vi "initialise.vi"(8 "error in (no error)":errorcluster, 11 "DAQ_DL091205Readers in":refnum<class "DAQ_DL091205Readers.lvclass">) -> (0 "error out":errorcluster, 3 "DAQ_DL091205Readers out":refnum<class "DAQ_DL091205Readers.lvclass">)   [LabVIEW 2010, in "DAQ_DL091205Readers.lvclass"]
doc: "The dynamic dispatch-version of this VI initalises the plug-in object by allocating and initalising any dynamic resources need."
uses:
  DAQ_DL091205Readers.lvclass
  DAQ_DL090211Scaffold/DAQ_DL090211Scaffold/DAQ_DL090211Scaffold.lvclass
  DAQ_DL091205Readers.lvclass/DAQ_DL091205Readers.ctl
  SignalReader/GenericSignalReader/GenericSignalReader/GenericSignalReader.lvclass
  common/classes/ErrorController/ErrorController/class_data.vi
  common/classes/ErrorController/ErrorController/ErrorController.lvclass
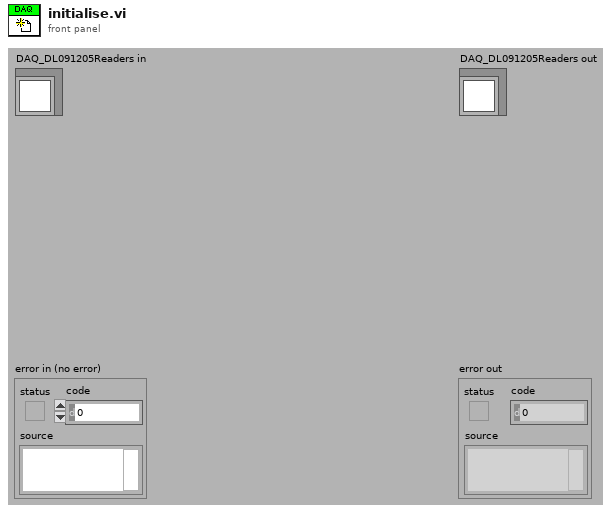
[diagram p1: front panel]
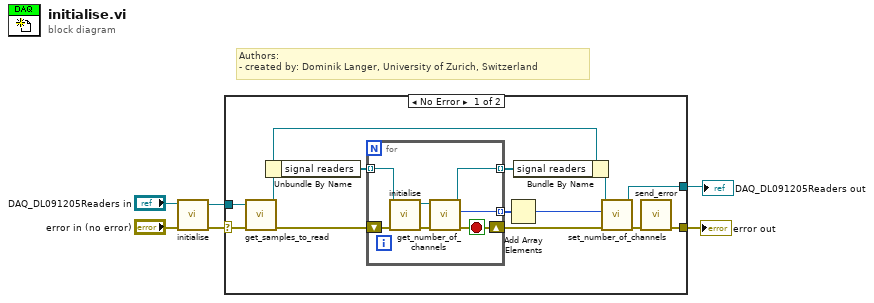
[diagram p0: block diagram]
diagram:
  # "Authors: \n- created by: Dominik Langer, University of Zurich, Switzerland"
  n1 = call-parent "initialise.vi"("error in (no error)"="error in (no error)", "GenericPlugin in"="DAQ_DL091205Readers in") -> ("error out"=w4:errorcluster, "GenericPlugin out"=w3:refnum<class "DAQ_DL091205Readers.lvclass">)  [unwired: 8 in]
  n2 = case shown="No Error" w4 {
    selector: w4 -> [w15 w27]
    tunnel: [w13 w27] -> w2
    tunnel: w3 -> [w17 w28]
    tunnel: [w8 w28] -> w1
    frame No Error {
      n3 = call-dynamic "get_samples_to_read.vi"("error in (no error)"=w15, "GenericDAQ.lvclass in"=w17) -> ("error out"=w14:errorcluster, "GenericDAQ.lvclass out"=w16:refnum<class "DAQ_DL091205Readers.lvclass">)  [unwired: 7 in, 1 out]
      n4 = Unbundle By Name(w16) -> ("signal readers"=w19:refnum<class "GenericSignalReader.lvclass">[])
      n5 = for {
        tunnel: w19 -> [w25] mode=indexing
        tunnel: [w21] -> w18 mode=indexing
        shift-right: [w23] -> w10
        shift-left: w14 -> [w26]
        tunnel: [w20] -> w12 mode=indexing
        stop <- w23 stop-if-true
        n6 = call-dynamic "initialise.vi"("error in (no error)"=w26, "GenericPlugin in"=w25) -> ("error out"=w24:errorcluster, "GenericPlugin out"=w22:refnum<class "GenericSignalReader.lvclass">)  [unwired: 8 in]
        n7 = call-dynamic "get_number_of_channels.vi"("error in (no error)"=w24, "GenericSignalReader in"=w22) -> ("error out"=w23:errorcluster, "number of channels"=w20:i32, "GenericSignalReader out"=w21:refnum<class "GenericSignalReader.lvclass">)  [unwired: 7 in]
      }
      n8 = Add Array Elements(numeric array=w12) -> (sum=w11:i32)
      n9 = Bundle By Name(cluster=w16, "signal readers"=w18) -> (w7:refnum<class "DAQ_DL091205Readers.lvclass">)
      n10 = call-dynamic "set_number_of_channels.vi"("error in (no error)"=w10, "number of channels"=w11, "GenericDAQ.lvclass in"=w7) -> ("error out"=w9:errorcluster, "GenericDAQ.lvclass out"=w8:refnum<class "DAQ_DL091205Readers.lvclass">)  [unwired: 7 in]
      n11 = call "send_error.vi"("error in (no error)"=w9) -> ("error out"=w13:errorcluster)  [unwired: 10 in]
    }
    frame Error {
    }
  }
  "error out" <- w2
  "DAQ_DL091205Readers out" <- w1
